vi "BRig_dataLC_ENL_PostR_Block_l1.vi"() -> (2 "output_ENL_PostR_Block":i32)   [LabVIEW 2014]
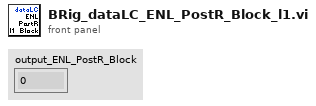
[diagram p1: front panel]
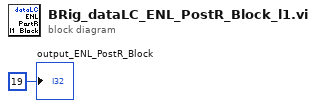
[diagram p0: block diagram]
diagram:
  "output_ENL_PostR_Block" <- 19 ("output_iBlock")
